vi "CSMLS - Continuous Loop in CSM Example.vi"() -> ()   [LabVIEW 2014]
uses:
  user.lib/_NEVSTOP/Communicable State Machine(CSM)/_Support/Priority Queue/Priority Queue.lvclass/Priority Queue.ctl
  user.lib/_NEVSTOP/Communicable State Machine(CSM)/_Support/Process/CSMP-Async Call.vi
  user.lib/_NEVSTOP/Communicable State Machine(CSM)/_Support/GlobalEvent/GEvt-Generate Status Log.vi
  user.lib/_NEVSTOP/Communicable State Machine(CSM)/_Support/Process/CSMP-Broadcast.vi
  user.lib/_NEVSTOP/Communicable State Machine(CSM)/_Support/GlobalEvent/GEvt-Generate Interrupt Log.vi
  user.lib/_NEVSTOP/Communicable State Machine(CSM)/_Support/GlobalEvent/GEvt-Generate Register Log.vi
  user.lib/_NEVSTOP/Communicable State Machine(CSM)/_Support/Process/CSMP-Register Status.vi
  user.lib/_NEVSTOP/Communicable State Machine(CSM)/_Support/GlobalEvent/GEvt-Generate Unregister Log.vi
  user.lib/_NEVSTOP/Communicable State Machine(CSM)/_Support/Process/CSMP-Unregister Status.vi
  user.lib/_NEVSTOP/Communicable State Machine(CSM)/_Support/Process/CSMP-Sync Call.vi
  user.lib/_NEVSTOP/Communicable State Machine(CSM)/_Support/CSMQ/_CSMObj-Unlock.vi
  user.lib/_NEVSTOP/Communicable State Machine(CSM)/_Support/Process/CSMP-PostPostMsg.vi
  user.lib/_NEVSTOP/Communicable State Machine(CSM)/_Support/Process/CSMP-PostSendMsg.vi
  user.lib/_NEVSTOP/Communicable State Machine(CSM)/_Support/CSMQ/_CSMObj-Lock State.vi
  user.lib/_NEVSTOP/Communicable State Machine(CSM)/_Support/Common/Splite Reason String Part.vi
  user.lib/_NEVSTOP/Communicable State Machine(CSM)/_Support/Common/Trim Single line Text.vi
  user.lib/_NEVSTOP/Communicable State Machine(CSM)/_Support/CSMQ/_CSMOFGV Release.vi
  user.lib/_NEVSTOP/Communicable State Machine(CSM)/_Support/Common/Remove Comments from Line.vi
  user.lib/_NEVSTOP/Communicable State Machine(CSM)/_Support/Common/Splite Single-line Message.vi
  user.lib/_NEVSTOP/Communicable State Machine(CSM)/_Support/Common/Parse Next Single-line State.vi
  user.lib/_NEVSTOP/Communicable State Machine(CSM)/_Support/CSMQ/_CSMOFGV Dequeue.vi
  user.lib/_NEVSTOP/Communicable State Machine(CSM)/_Support/CSMQ/_CSMObj-Log Error if in a Remote Session.vi
  user.lib/_NEVSTOP/Communicable State Machine(CSM)/_Support/GlobalEvent/GEvt-Generate State Change Log.vi
  user.lib/_NEVSTOP/Communicable State Machine(CSM)/_Support/GlobalEvent/GEvt-Generate Remaining States Log.vi
  user.lib/_NEVSTOP/Communicable State Machine(CSM)/_Support/GlobalEvent/GEvt-Generate Module Destroyed Log.vi
  user.lib/_NEVSTOP/Communicable State Machine(CSM)/_Support/GlobalEvent/GEvt-Generate Complete Log.vi
  user.lib/_NEVSTOP/Communicable State Machine(CSM)/_Support/GlobalEvent/GEvt-Generate Module Created Log.vi
  user.lib/_NEVSTOP/Communicable State Machine(CSM)/AdvanceAPI/CSM - Revert Arguments-Safe String.vi
  user.lib/_NEVSTOP/Communicable State Machine(CSM)/AdvanceAPI/CSM - Make String Arguments Safe.vi
  user.lib/_NEVSTOP/Communicable State Machine(CSM)/_Support/CSMQ/_CSMObj-Message Check.vi
  user.lib/_NEVSTOP/Communicable State Machine(CSM)/_Support/CSMQ/_CSMObj-Enqueue Cross-Module Message.vi
  user.lib/_NEVSTOP/Communicable State Machine(CSM)/_Support/CSMQ/_CSMOFGV Get.vi
  user.lib/_NEVSTOP/Communicable State Machine(CSM)/_Support/FGV-BroadcastRegistry/Cache-Broadcast Registry Search Result.vi
  user.lib/_NEVSTOP/Communicable State Machine(CSM)/AdvanceAPI/CSM - Register Status Change.vi
  user.lib/_NEVSTOP/Communicable State Machine(CSM)/AdvanceAPI/CSM - Unregister Status Change.vi
  user.lib/_NEVSTOP/Communicable State Machine(CSM)/_Support/Common/Hex Str to U8 Data.vi
  user.lib/_NEVSTOP/Communicable State Machine(CSM)/_Support/Common/Concatenate State with Arguments.vi
  user.lib/_NEVSTOP/Communicable State Machine(CSM)/_Support/Common/U8 Data to Hex Str.vi
  user.lib/_NEVSTOP/Communicable State Machine(CSM)/_Support/Priority Queue/Dequeue Element.vi
  user.lib/_NEVSTOP/Communicable State Machine(CSM)/AdvanceAPI/CSM - Keywords.vi
  user.lib/_NEVSTOP/Communicable State Machine(CSM)/_Support/Priority Queue/Enqueue Element.vi
  user.lib/_NEVSTOP/Communicable State Machine(CSM)/Utility/Trim Both Whitespace.vi
  user.lib/_NEVSTOP/Communicable State Machine(CSM)/_Support/GlobalEvent/FGV-GlobalEventRef.vi
  user.lib/_NEVSTOP/Communicable State Machine(CSM)/_Support/CSMQ/_CSMOFGV Obtain.vi
  user.lib/_NEVSTOP/Communicable State Machine(CSM)/_Support/CSMQ/_CSMOFGV.vi
  user.lib/_NEVSTOP/Communicable State Machine(CSM)/_Support/GlobalEvent/FGV-StatusChangeEventRef.vi
  user.lib/_NEVSTOP/Communicable State Machine(CSM)/_Support/FGV-BroadcastRegistry/global-Broadcast Cache Change Flag.vi
  user.lib/_NEVSTOP/Communicable State Machine(CSM)/_Support/FGV-BroadcastRegistry/FGV-BroadcastRegistry.vi
  user.lib/_NEVSTOP/Communicable State Machine(CSM)/Communicable State Machine.lvlib
  user.lib/_NEVSTOP/Communicable State Machine(CSM)/addons/Loop-Support/CSM Loop Support.lvlib
panel:
  in  "High-Priority Error":bool
  in  "Low-Priority Error":bool
  out "Filtered UI States":string
  out "UI States":string
  out ">> Source CSM >>":string
  out "Remaining States":string
  in  "DAQ: Once":bool
  out "Waveform Chart":dbl(graph)=7.7472539242125515
  in  "Center":dbl(slide) scale=0.0..10.0
  in  "Stop":bool
  in  "Start":bool
  out "State History":string
  in  "Name(\"\" to use uuid)":string="CSM Tiny"
  in  "Init State(\"Macro: Initialize\")":string="Macro: Initialize"
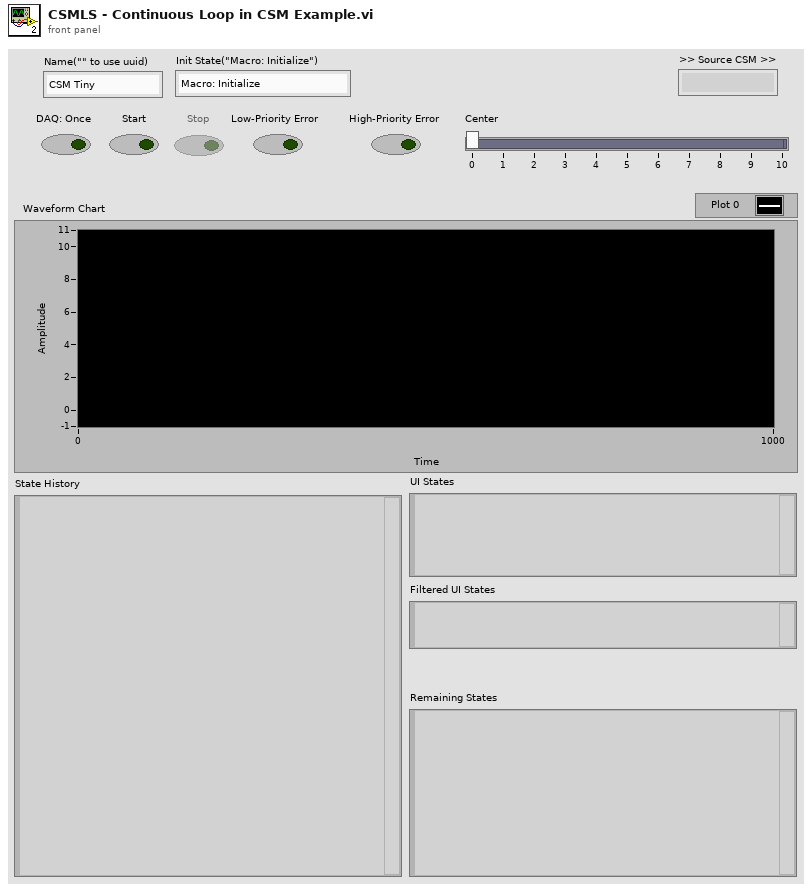
[diagram p1: front panel]
types:
  T1 = enum32{"Invalid", "Standard", "Closed", "Hidden", "Minimized", "Maximized"}
  T2 = enum32{"invalid app kind", "Development System", "Run Time System", "Student Edition", "Embedded LabVIEW", "Evaluation", "Custom"}
  T3 = typedef "Communicable State Machine.lvlib/_CSM_Response Source Message.ctl" = cluster{"‘State":string, "’Arguments":string, "’Error":errorcluster}
  T4 = cluster{"Core":cluster{"Current VI Reference":refnum<vi>, "Close Panel on Exit?":bool}, "IsRunning?":bool, "Center":dbl}
  T5 = cluster{"Current VI Reference":refnum<vi>, "Close Panel on Exit?":bool}
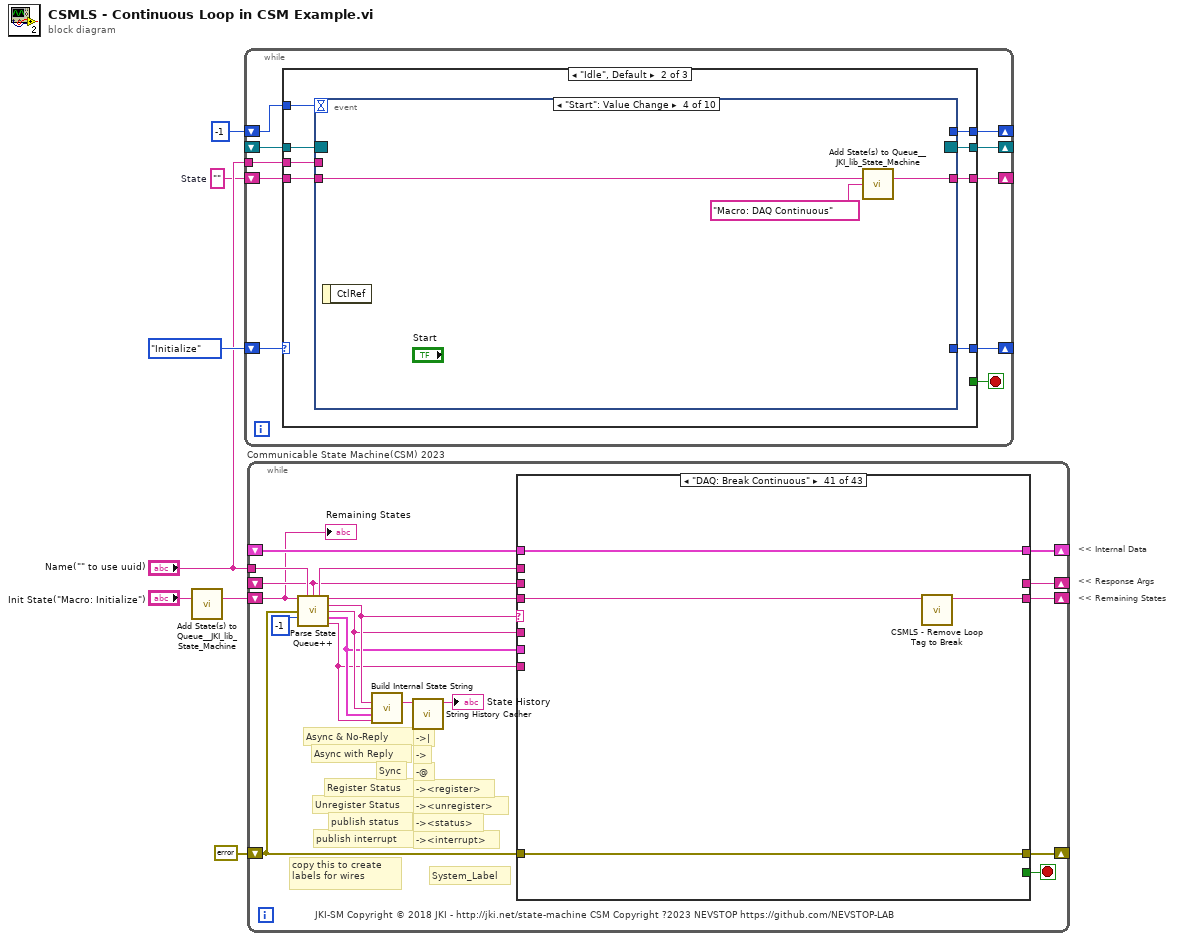
[diagram p0: block diagram]
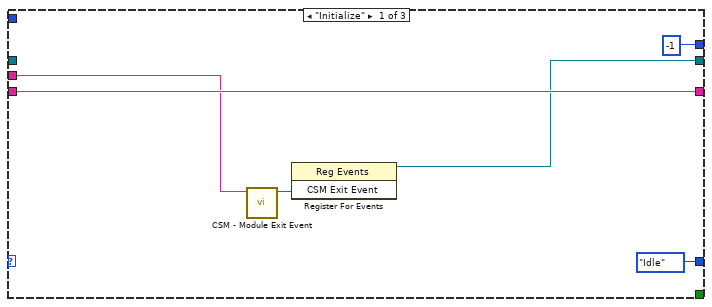
[diagram p2: hidden frame]
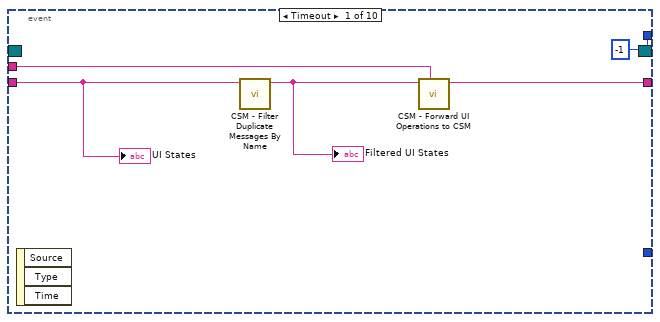
[diagram p3: hidden frame]
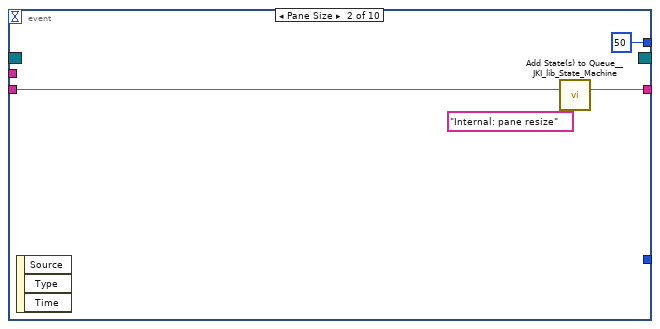
[diagram p4: hidden frame]
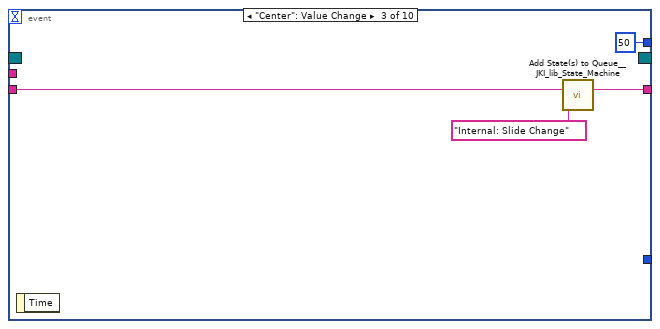
[diagram p5: hidden frame]
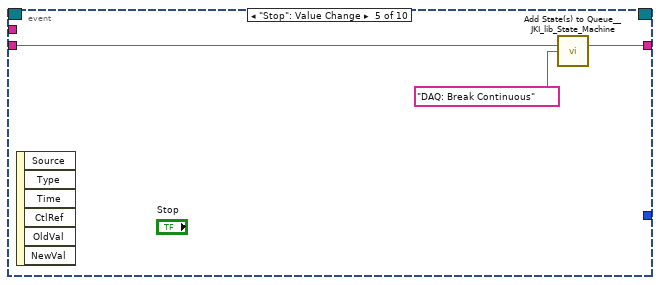
[diagram p6: hidden frame]
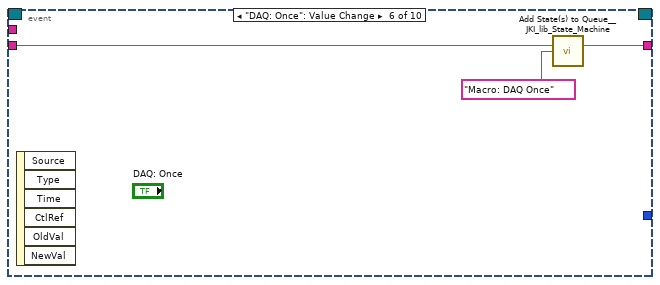
[diagram p7: hidden frame]
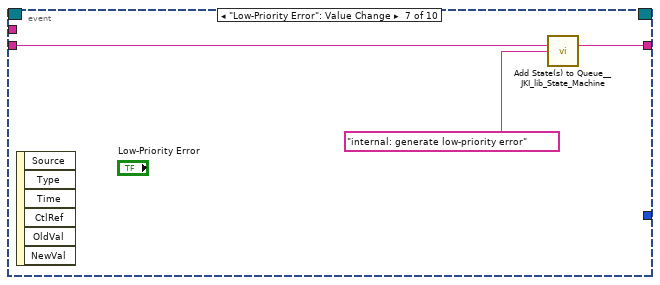
[diagram p8: hidden frame]
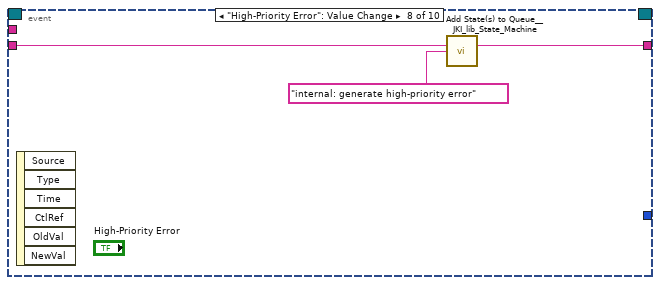
[diagram p9: hidden frame]
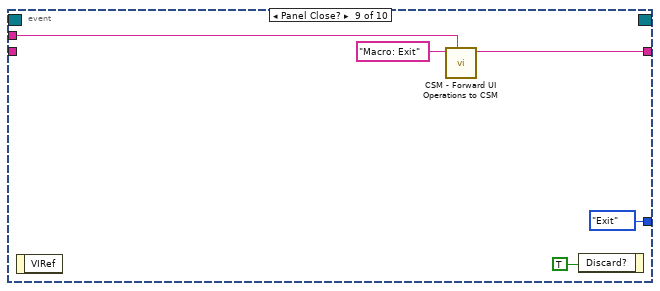
[diagram p10: hidden frame]
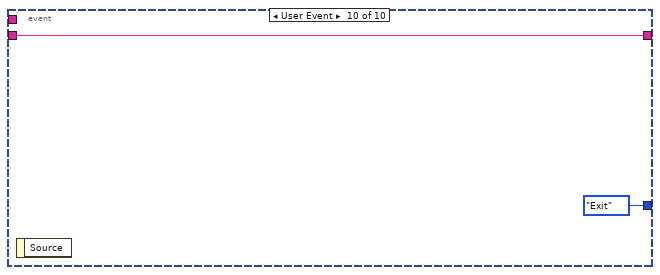
[diagram p11: hidden frame]
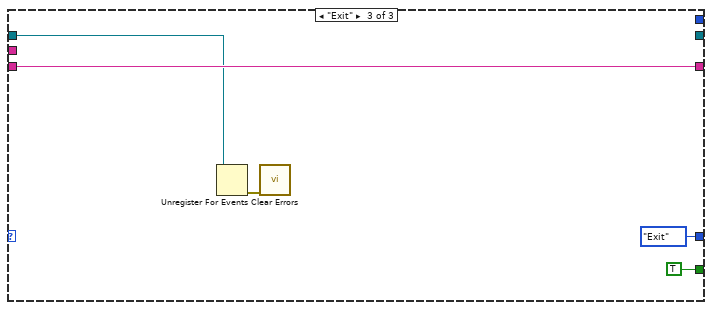
[diagram p12: hidden frame]
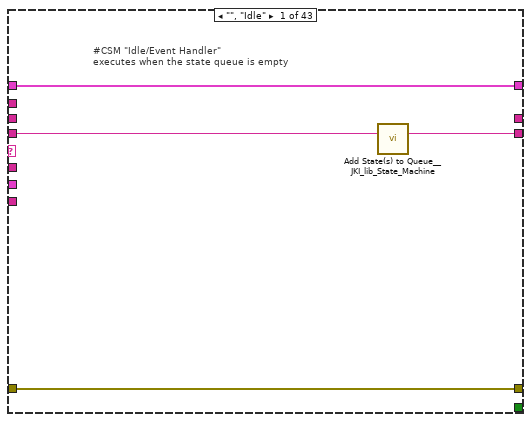
[diagram p13: hidden frame]
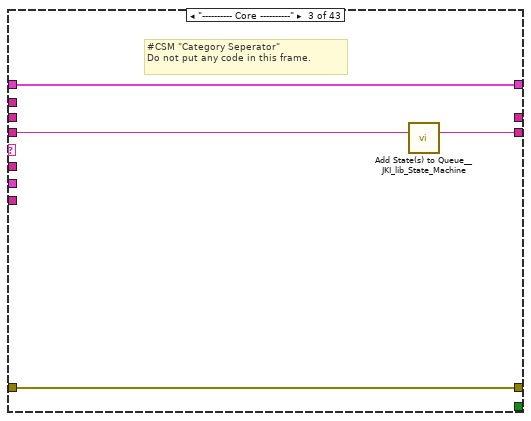
[diagram p15: hidden frame]
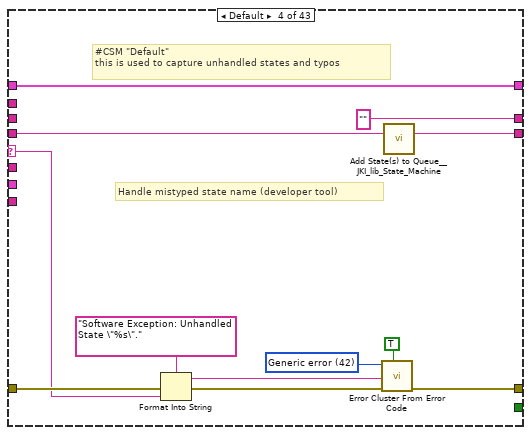
[diagram p16: hidden frame]
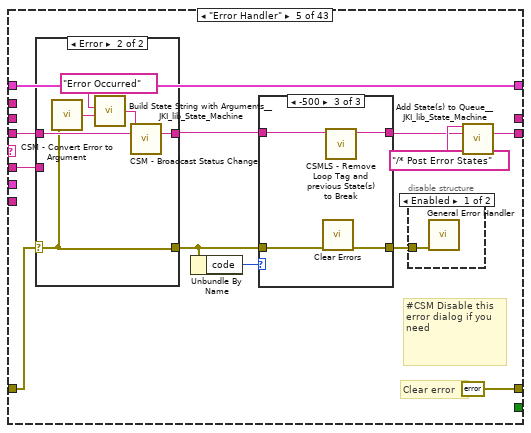
[diagram p17: hidden frame]
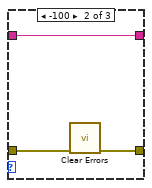
[diagram p19: hidden frame]
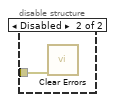
[diagram p20: hidden frame]
diagram:
  w2 = ""  # State
  # "<< Internal Data"
  # "<< Response Args"
  # "<< Remaining States"
  n1 = call <vilib>:"Add State(s) to Queue__JKI_lib_State_Machine.vi"("State(s) in (\"\")"="Init State(\"Macro: Initialize\")") -> ("States Out"=w5:string)  [unwired: 14 in]
  n2 = while {
    shift-right: [w16] -> _
    shift-left: enum16{"Idle", "Initialize", "Exit"}."Initialize" -> [w17]
    tunnel: "Name(\"\" to use uuid)" -> [w14]
    shift-right: [w12] -> _
    shift-left: w2 -> [w13]
    shift-right: [w10] -> _
    shift-left: -1 -> [w11]
    shift-right: [w9] -> _
    shift-left: _ -> [w8]
    stop <- w15 stop-if-true
    n3 = case shown="\"Idle\", Default" w17 {
      tunnel: [enum16{"Idle", "Initialize", "Exit"}."Idle" w31 enum16{"Idle", "Initialize", "Exit"}."Exit"] -> w16
      tunnel: [_ _ TRUE] -> w15
      tunnel: w14 -> [w19 w30 _]
      tunnel: w13 -> [w22 w28 w69]
      tunnel: [w22 w29 w69] -> w12
      tunnel: w11 -> [_ w26 _]
      tunnel: [-1 w27 _] -> w10
      tunnel: [w18 w24 _] -> w9
      tunnel: w8 -> [_ w25 w68]
      frame "Initialize" {
        n4 = call "CSM - Module Exit Event.vi"("Name(\"\" to use uuid) in"=w19) -> ("CSM Exit Event"=w20:refnum<user-event>)  [unwired: 9 in, 1 out]
        n5 = register-events(w20) -> (reference out=w18:refnum<event-registration>)  [unwired: 2 in, 1 out]
      }
      frame "Idle", Default {
        n6 = event shown="[3] \"Start\": Value Change" {
          selector: w25 -> [_ _ _ _ _ _ _ _ _ _]
          dyn-events: [_ _ _ _ _ _ _ _ _ _] -> w24
          timeout: w26 -> [_ _ _ _ _ _ _ _ _ _]
          tunnel: [_ _ _ _ _ _ _ _ enum16{"Idle", "Initialize", "Exit"}."Exit" enum16{"Idle", "Initialize", "Exit"}."Exit"] -> w31
          tunnel: w30 -> [w32 _ _ _ _ _ _ _ w61 _]
          tunnel: w28 -> [w35 w40 w44 w47 w49 w52 w56 w58 _ w66]
          tunnel: [w33 w39 w43 w46 w50 w53 w55 w57 w60 w66] -> w29
          tunnel: [-1 50 50 _ _ _ _ _ _ _] -> w27
          event Timeout {
            n7 = event-data() -> ()  [unwired: 1 in, 3 out]
            n8 = call "CSM - Filter Duplicate Messages By Name.vi"("States"=w35) -> ("States out"=w34:string)  [unwired: 10 in]
            "Filtered UI States" <- w34
            n9 = call "CSM - Forward UI Operations to CSM.vi"("Name(\"\" to use uuid)"=w32, "State(s) in (\"\")"=w34) -> ("States Out"=w33:string)  [unwired: 9 in]
            "UI States" <- w35
          }
          event Pane Size {
            n10 = event-data() -> ()  [unwired: 1 in, 3 out]
            n11 = call <vilib>:"Add State(s) to Queue__JKI_lib_State_Machine.vi"("State(s) in (\"\")"=w40, "State(s) at Back (\"\")"="Internal: pane resize" ("State(s) at Back (\"\")")) -> ("States Out"=w39:string)  [unwired: 13 in]
          }
          event "Center": Value Change {
            n12 = event-data() -> ()  [unwired: 1 in, 1 out]
            n13 = call <vilib>:"Add State(s) to Queue__JKI_lib_State_Machine.vi"("State(s) in (\"\")"=w44, "State(s) at Back (\"\")"="Internal: Slide Change" ("State(s) at Back (\"\")")) -> ("States Out"=w43:string)  [unwired: 13 in]
          }
          event "Start": Value Change {
            n14 = event-data() -> ()  [unwired: 1 in, 1 out]
            n15 = call <vilib>:"Add State(s) to Queue__JKI_lib_State_Machine.vi"("State(s) in (\"\")"=w47, "State(s) at Back (\"\")"="Macro: DAQ Continuous" ("State(s) at Back (\"\")")) -> ("States Out"=w46:string)  [unwired: 13 in]
          }
          event "Stop": Value Change {
            n16 = event-data() -> ()  [unwired: 1 in, 6 out]
            n17 = call <vilib>:"Add State(s) to Queue__JKI_lib_State_Machine.vi"("State(s) in (\"\")"=w49, "State(s) at Back (\"\")"="DAQ: Break Continuous" ("State(s) at Back (\"\")")) -> ("States Out"=w50:string)  [unwired: 13 in]
          }
          event "DAQ: Once": Value Change {
            n18 = event-data() -> ()  [unwired: 1 in, 6 out]
            n19 = call <vilib>:"Add State(s) to Queue__JKI_lib_State_Machine.vi"("State(s) in (\"\")"=w52, "State(s) at Back (\"\")"="Macro: DAQ Once" ("State(s) at Back (\"\")")) -> ("States Out"=w53:string)  [unwired: 13 in]
          }
          event "Low-Priority Error": Value Change {
            n20 = event-data() -> ()  [unwired: 1 in, 6 out]
            n21 = call <vilib>:"Add State(s) to Queue__JKI_lib_State_Machine.vi"("State(s) in (\"\")"=w56, "State(s) at Back (\"\")"="internal: generate low-priority error" ("State(s) at Back (\"\")")) -> ("States Out"=w55:string)  [unwired: 13 in]
          }
          event "High-Priority Error": Value Change {
            n22 = event-data() -> ()  [unwired: 1 in, 6 out]
            n23 = call <vilib>:"Add State(s) to Queue__JKI_lib_State_Machine.vi"("State(s) in (\"\")"=w58, "State(s) at Back (\"\")"="internal: generate high-priority error" ("State(s) at Back (\"\")")) -> ("States Out"=w57:string)  [unwired: 13 in]
          }
          event Panel Close? {
            n24 = event-data() -> ()  [unwired: 1 in, 1 out]
            n25 = call "CSM - Forward UI Operations to CSM.vi"("Name(\"\" to use uuid)"=w61, "State(s) in (\"\")"="Macro: Exit" ("State")) -> ("States Out"=w60:string)  [unwired: 9 in]
            n26 = event-data("Discard?"=TRUE) -> ()  [unwired: 1 in, 1 out]
          }
          event User Event {
            n27 = event-data() -> ()  [unwired: 1 in, 1 out]
          }
        }
      }
      frame "Exit" {
        n28 = Unregister For Events(event registration refnum=w68) -> (error out=w67:errorcluster)  [unwired: 1 in]
        n29 = call <vilib>:"Clear Errors.vi"("error in (no error)"=w67) -> ()  [unwired: 5 in, 2 out]
      }
    }
  }
  n30 = while "Communicable State Machine(CSM) 2023" {
    shift-right: [w86] -> _
    shift-left: _ -> [w85]
    shift-right: [w89] -> _
    shift-left: errorcluster {"status"=FALSE, "code"=0, "source"=""} ("error out") -> [w84]
    shift-right: [w88] -> _
    shift-left: w5 -> [w72]
    tunnel: "Name(\"\" to use uuid)" -> [w82]
    shift-right: [w83] -> _
    shift-left: _ -> [w74]
    stop <- w87 stop-if-true
    # "-><interrupt>"
    # "-><status>"
    # "-><unregister>"
    # "-><register>"
    # "-@"
    # "->"
    # "->|"
    # "publish interrupt"
    # "publish status"
    # "Unregister Status"
    # "Register Status"
    # "Sync"
    # "Async with Reply"
    # "Async & No-Reply"
    # "copy this to create labels for wires"
    # "System_Label"
    # "JKI-SM Copyright © 2018 JKI - http://jki.net/state-machine CSM Copyright ?2023 NEVSTOP https://github.com/NEVSTOP-LAB"
    n31 = call "Parse State Queue++.vi"("State Queue"=w72, "Name(\"\" to use uuid)"=w82, "Response Arguments"=w74, "Error In (no error)"=w84, "Dequeue Timeout(0ms)"=-1 ("Timeout")) -> ("Name Used"=w75:string, "Remaining States"=w90:string, "Current State"=w79:string, "Arguments"=w78:string, ">> Response Source Message >>"=w77:T3, ">> Source CSM >>"=w76:string)  [unwired: 5 in]
    n32 = call "Build Internal State String.vi"("State"=w79, "Arguments (\"\")"=w78, ">> Response Source Message >>"=w77, "Source (\"\")"=w76) -> ("State with Arguments"=w80:string)  [unwired: 11 in]
    n33 = call "String History Cacher.vi"("String"=w80) -> ("String Cache"=→"State History":string)  [unwired: 10 in]
    n34 = case shown="\"DAQ: Break Continuous\"" w79 {
      selector: w79 -> [_ _ _ w103 _ _ w160 _ _ _ _ _ _ _ _ _ _ _ _ _ _ _ _ _ _ _ _ _ _ _ _ _ _ _ _ _ _ _ _ w417 _ _ _]
      tunnel: w90 -> [w91 w96 w101 w107 w122 w154 w162 w172 w183 w197 w202 w206 w213 w215 w222 w226 w232 w238 w253 w331 w336 w341 w343 w348 w352 w360 w364 w369 w376 w380 w384 w388 w392 w395 w397 w400 w403 w408 w414 w419 w425 w431 w434]
      tunnel: w78 -> [_ _ _ _ w121 w147 w161 w171 _ _ _ _ _ _ _ _ _ w233 w247 _ _ _ _ _ _ _ _ w367 _ _ _ _ _ _ _ _ _ _ _ _ _ _ _]
      tunnel: w85 -> [w92 w95 w98 w105 w124 w155 w163 w174 w182 w190 w200 w203 _ w214 w217 w223 w230 w236 w249 w330 w333 w338 w345 w350 w354 w359 w363 w368 w373 w377 w381 w387 w391 w394 w396 w399 w402 w407 w411 w422 w426 w430 w433]
      tunnel: [w93 w97 w99 w109 errorcluster {"status"=FALSE, "code"=0, "source"=""} ("error out") w156 w158 w177 w184 w194 w199 w204 w210 w216 w218 w224 w229 w234 w250 w332 w334 w339 w346 w351 w357 w361 w365 w370 w374 w378 w382 w389 errorcluster {"status"=TRUE, "code"=-100, "source"="Low priority error. Daq could continue."} ("error out") errorcluster {"status"=TRUE, "code"=-500, "source"="High priority error. Daq need stop!"} ("error out") w398 w401 w404 w409 w415 w423 w427 w432 w435] -> w89
      tunnel: w84 -> [w93 w97 w99 w108 w123 w156 w165 _ w184 w194 w199 w204 w210 w216 w219 w224 w229 w235 w251 w332 w334 w339 w346 w351 w357 w361 w365 w370 w374 w378 w382 w389 _ _ w398 w401 w404 w409 w415 w423 w427 w432 w435]
      tunnel: [w94 w96 w100 w106 w119 w153 w164 w173 w183 w196 w201 w205 w212 w215 w221 w225 w231 w237 w252 w331 w335 w340 w344 w349 w358 w360 w364 w369 w375 w379 w383 w388 w392 w395 w397 w400 w403 w408 w414 w420 w424 w431 w434] -> w88
      tunnel: [_ _ _ _ _ TRUE _ _ _ _ TRUE _ _ _ _ _ _ _ _ _ _ _ _ _ _ _ _ _ _ _ _ _ _ _ _ _ _ _ _ _ _ _ _] -> w87
      tunnel: [w92 w95 w98 w105 w124 w155 w163 w175 w182 w195 w200 w203 w211 w214 w217 w223 w230 w236 w249 w330 w333 w338 w345 w350 w354 w359 w363 w368 w373 w377 w381 w386 w391 w394 w396 w399 w402 w406 w411 w422 w426 w429 w433] -> w86
      tunnel: w76 -> [_ _ _ _ _ _ _ w169 _ _ _ _ _ _ _ _ _ _ _ _ _ _ _ _ _ _ _ _ _ _ _ _ _ _ _ _ _ _ _ w418 _ _ _]
      tunnel: w77 -> [_ _ _ _ _ _ _ w176 _ _ _ _ _ _ _ _ _ _ _ _ _ _ _ _ _ _ _ _ _ _ _ _ _ _ _ _ _ _ _ _ _ _ _]
      tunnel: [_ _ _ "" _ _ _ _ _ _ _ _ _ _ _ _ _ _ _ _ _ _ _ _ _ _ "API1 Response" w366 _ _ _ _ _ _ _ _ _ _ _ _ _ _ _] -> w83
      tunnel: w75 -> [_ _ _ _ _ _ _ _ _ _ _ _ _ _ _ _ _ _ _ _ _ _ _ _ _ _ _ _ _ _ _ _ _ _ _ _ _ _ _ _ _ _ _]
      tunnel: w74 -> [_ _ _ _ _ _ _ _ _ _ _ _ _ _ _ _ _ _ _ _ _ _ _ _ _ _ _ _ _ _ _ _ _ _ _ _ _ _ _ _ _ _ _]
      frame "", "Idle" {
        # "#CSM \"Idle/Event Handler\"\nexecutes when the state queue is empty"
        n35 = call <vilib>:"Add State(s) to Queue__JKI_lib_State_Machine.vi"("State(s) in (\"\")"=w91) -> ("States Out"=w94:string)  [unwired: 14 in]
      }
      frame "CSM Documentation" {
        # "#CSM README FIRST\n\nCSM is a LabVIEW application framework that builds upon JKI State Machine (JKISM). It follows the pattern of JKISM and extends the keywords to describe message communication between CSM modules, including concepts such as Sync-Message, Async-Message, Subscription/Unsubscription of status - essential elements for creating reusable code modules. For more information, please visit the CSM wiki: https://github.com/NEVSTOP-LAB/JKI-State-Machine-Plus-Plus/wiki\n\nFor instructions on JKI State Machine, visit: http://jki.net/state-machine/\nFor information about CSM, visit: https://github.com/NEVSTOP-LAB"
        # "#CSM \"Documentation\"\nCase for holding CSM Documenation"
      }
      frame "---------- Core ----------" {
        # "#CSM \"Category Seperator\"\nDo not put any code in this frame."
        n36 = call <vilib>:"Add State(s) to Queue__JKI_lib_State_Machine.vi"("State(s) in (\"\")"=w101) -> ("States Out"=w100:string)  [unwired: 14 in]
      }
      frame Default {
        w112 = 42 items=["No error", "Argument error", "Memory is full", "Out of zone", "End of file", "File already open", "Generic file I/O error", "File not found", "File permission error", "Disk is full", "Duplicate path", "Too many files open", "System feature not enabled", "Resource file not found", "Cannot add resource", "Resource not found", "Image not found", "Image memory error", "Pen does not exist", "Config type invalid", "Config token not found", "Config parse error", "Config memory error", "Bad external code format", "Bad external code offset", "External code not present", "Null window", "Destroy window error", "Null menu", "Print aborted", "Bad print record", "Print driver error", "Windows error during printing", "Memory error during printing", "Print dialog error", "Generic print error", "Invalid device refnum", "Device not found", "Device parameter error", "Device unit error", "Cannot open device", "Device call aborted", "Generic error", "Cancelled by user", "Object ID too low", "Object ID too high", "Object not in heap", "Unknown heap", "Unknown object (invalid DefProc)", "Unknown object (DefProc not in table)", "Message out of range", "Invalid (null) method", "Unknown message", "Manager call not supported", "Bad address", "Network operation in progress", "Network operation timed out", "Connection is busy", "Network attribute not supported", "Network error", "Address in use", "System out of memory", "Connection aborted", "Connection refused", "Not connected", "Already connected", "Connection closed", "Initialization error (interapplication manager)", "Bad occurrence", "Wait on unbound occurrence handler", "Occurrence queue overflow", "Datalog type conflict", "Unused", "Unrecognized type (interapplication manager)", "Memory corrupt", "Failed to make temporary DLL", "Old CIN version", "Drag socket not found", "Failed to load drop-object", "Failed to register OLE object", "Failed to release OLE object", "Format specifier type mismatch", "Unknown format specifier", "Too few format specifiers", "Too many format specifiers", "Scan failed", "Newer CIN version", "Error converting to variant", "Runtime menu error", "Password tampered", "Variant attribute not found", "Incompatible variant data type", "Event data is not available", "Event Store is not present", "Occurrence is not found", "Event Queue is not created", "Event info is not available", "Refnum passed is NULL", "Error retrieving Class GUID", "Error retrieving CoClass GUID", "Error retrieving TypeLib GUID.", "Bad built application magic bytes.", "Specific driver is different from the specific driver associated with the Logical Name.", "There is no session opened to the class driver.", "Max Error", "MAX - Error with config objects", "MAX - Error loading configuration", "MAX - Group not supported"]
        # "#CSM \"Default\"\nthis is used to capture unhandled states and typos"
        # "Handle mistyped state name (developer tool)"
        n37 = Format Into String(format string="Software Exception: Unhandled State \"%s\"." ("message"), error in=w108, w103) -> (resulting string=w111:string, error out=w110:errorcluster)  [unwired: 1 in]
        n38 = call <vilib>:"Error Cluster From Error Code.vi"("show call chain? (False)"=TRUE, "error in (no error)"=w110, "error message (\"\")"=w111, "error code (0)"=w112) -> ("error out"=w109:errorcluster)  [unwired: 5 in]
        n39 = call <vilib>:"Add State(s) to Queue__JKI_lib_State_Machine.vi"("State(s) in (\"\")"=w107) -> ("States Out"=w106:string)  [unwired: 14 in]
      }
      frame "Error Handler" {
        # "#CSM Disable this error dialog if you need"
        # "Clear error"
        n40 = case shown="Error" w123 {
          selector: w123 -> [_ w140]
          tunnel: [w139 w141] -> w114
          tunnel: w122 -> [w139 w142]
          tunnel: w121 -> [w138 _]
          tunnel: [w137 w140] -> w117
          frame No Error {
            n41 = call "CSM - Convert Argument to Error.vi"("Argument"=w138) -> ("error"=w137:errorcluster)  [unwired: 4 in]
          }
          frame Error {
            n42 = call "CSM - Convert Error to Argument.vi"("error in (no error)"=w140) -> ("Arguments"=w144:string)  [unwired: 4 in]
            n43 = call <vilib>:"Build State String with Arguments__JKI_lib_State_Machine.vi"("Arguments (\"\")"=w144, "State"="Error Occurred" ("Status with Arguments")) -> ("State with Arguments"=w143:string)  [unwired: 4 in]
            n44 = call "CSM - Broadcast Status Change.vi"("Status with Arguments"=w143, "State Queue"=w142) -> ("Remaining States"=w141:string)  [unwired: 13 in]
          }
        }
        n45 = Unbundle By Name(w117) -> ("code"=w118:i32)
        n46 = case shown="-500" w118 {
          tunnel: w117 -> [w127 w130 w134]
          tunnel: [w127 w129 w131] -> w116
          tunnel: [w126 w128 w132] -> w115
          tunnel: w114 -> [w126 w128 w133]
          frame 0, Default {
          }
          frame -100 {
            n47 = call <vilib>:"Clear Errors.vi"("error in (no error)"=w130) -> ("error out"=w129:errorcluster)  [unwired: 5 in, 1 out]
          }
          frame -500 {
            n48 = call <vilib>:"Clear Errors.vi"("error in (no error)"=w134) -> ("error out"=w131:errorcluster)  [unwired: 5 in, 1 out]
            n49 = call "CSMLS - Remove Loop Tag and previous State(s) to Break.vi"("Remaining States"=w133) -> ("States"=w132:string)  [unwired: 10 in]
          }
        }
        n50 = disable-structure shown="Enabled" {
          disable-tunnel: w116 -> [w135 w136]
          frame Enabled {
            n51 = call <vilib>:"General Error Handler.vi"("error in (no error)"=w135) -> ()  [unwired: 10 in, 5 out]
          }
          frame Disabled {
            n52 = call <vilib>:"Clear Errors.vi"("error in (no error)"=w136) -> ()  [unwired: 5 in, 2 out]
          }
        }
        n53 = call <vilib>:"Add State(s) to Queue__JKI_lib_State_Machine.vi"("State(s) in Front (\"\")"="/* Post Error States", "State(s) in (\"\")"=w115) -> ("States Out"=w119:string)  [unwired: 13 in]
      }
      frame "Critical Error" {
        w151 = 42 items=["No error", "Argument error", "Memory is full", "Out of zone", "End of file", "File already open", "Generic file I/O error", "File not found", "File permission error", "Disk is full", "Duplicate path", "Too many files open", "System feature not enabled", "Resource file not found", "Cannot add resource", "Resource not found", "Image not found", "Image memory error", "Pen does not exist", "Config type invalid", "Config token not found", "Config parse error", "Config memory error", "Bad external code format", "Bad external code offset", "External code not present", "Null window", "Destroy window error", "Null menu", "Print aborted", "Bad print record", "Print driver error", "Windows error during printing", "Memory error during printing", "Print dialog error", "Generic print error", "Invalid device refnum", "Device not found", "Device parameter error", "Device unit error", "Cannot open device", "Device call aborted", "Generic error", "Cancelled by user", "Object ID too low", "Object ID too high", "Object not in heap", "Unknown heap", "Unknown object (invalid DefProc)", "Unknown object (DefProc not in table)", "Message out of range", "Invalid (null) method", "Unknown message", "Manager call not supported", "Bad address", "Network operation in progress", "Network operation timed out", "Connection is busy", "Network attribute not supported", "Network error", "Address in use", "System out of memory", "Connection aborted", "Connection refused", "Not connected", "Already connected", "Connection closed", "Initialization error (interapplication manager)", "Bad occurrence", "Wait on unbound occurrence handler", "Occurrence queue overflow", "Datalog type conflict", "Unused", "Unrecognized type (interapplication manager)", "Memory corrupt", "Failed to make temporary DLL", "Old CIN version", "Drag socket not found", "Failed to load drop-object", "Failed to register OLE object", "Failed to release OLE object", "Format specifier type mismatch", "Unknown format specifier", "Too few format specifiers", "Too many format specifiers", "Scan failed", "Newer CIN version", "Error converting to variant", "Runtime menu error", "Password tampered", "Variant attribute not found", "Incompatible variant data type", "Event data is not available", "Event Store is not present", "Occurrence is not found", "Event Queue is not created", "Event info is not available", "Refnum passed is NULL", "Error retrieving Class GUID", "Error retrieving CoClass GUID", "Error retrieving TypeLib GUID.", "Bad built application magic bytes.", "Specific driver is different from the specific driver associated with the Logical Name.", "There is no session opened to the class driver.", "Max Error", "MAX - Error with config objects", "MAX - Error loading configuration", "MAX - Group not supported"]
        # "#CSM Stop in Critical Error\nWhen Critical Error occurs, Stop the loop immediately. Do NOT change this unless you fully understand the impact."
        # "#CSM \"Critical Error\"\nWhen any un-recoverable error occurs, CSM goes into this case."
        # "Handle mistyped state name (developer tool)"
        n54 = Format Into String(format string="Software Exception: Critical Error\"%s\"." ("message"), w147) -> (resulting string=w150:string, error out=w149:errorcluster)  [unwired: 2 in]
        n55 = call <vilib>:"Error Cluster From Error Code.vi"("show call chain? (False)"=TRUE, "error in (no error)"=w149, "error message (\"\")"=w150, "error code (0)"=w151) -> ()  [unwired: 5 in, 1 out]
        n56 = call <vilib>:"Add State(s) to Queue__JKI_lib_State_Machine.vi"("State(s) in (\"\")"=w154) -> ("States Out"=w153:string)  [unwired: 14 in]
      }
      frame "Target Error", "Target Timeout Error" {
        # "#CSM \"Target Error\"\nWhen This CSM try to communicate with an un-existed CSM, This CSM goes into this case."
        # "#CSM \"Target Timeout Error\"\nWhen This CSM could not get the sync-call response in time, This CSM goes into this case."
        n57 = Format Into String(format string="Software Exception: %s now \"%s\"." ("message"), error in=w165, w160, w161) -> (resulting string=w159:string)  [unwired: 1 in, 1 out]
        n58 = call "Build Error Cluster.vi"("String to Prepend to source (\"\")"=w159, "code"=-1) -> ("error out"=w158:errorcluster)
        n59 = call <vilib>:"Add State(s) to Queue__JKI_lib_State_Machine.vi"("State(s) in (\"\")"=w162) -> ("States Out"=w164:string)  [unwired: 14 in]
      }
      frame "Async Response", "Response" {
        n60 = Unbundle(w176) -> ("‘State"=w170:string, "’Arguments"=w168:string, "’Error"=w167:errorcluster)
        n61 = case shown="Default" w170 {
          tunnel: [w181] -> w177
          tunnel: w167 -> [w181]
          tunnel: [w180] -> w175
          tunnel: w174 -> [w180]
          tunnel: [w178] -> w173
          tunnel: w172 -> [w179]
          tunnel: w171 -> [_]
          tunnel: w169 -> [_]
          tunnel: w168 -> [_]
          frame Default {
            # "#CSM Response Comments\nAfter Message is executed, CSM goes to this state for receive the response.\n    For Async Message(->), \"Async Response\" is used. This CSM will goes to \"Async Message Posted\" immediately and receive the \"Async Response\" after the callee finishes the message.\n    For Sync Message(@),  This CSM will wait until the message is done and immediately goes to \"Response\""
            # "#CSM \"Async Response\"\nHandle Async-call Response (\"Async Response\" for ->)"
            # "#CSM \"Response\"\nHandle Sync-call Response (\"Response\" for -@)"
            n62 = call <vilib>:"Add State(s) to Queue__JKI_lib_State_Machine.vi"("State(s) in (\"\")"=w179) -> ("States Out"=w178:string)  [unwired: 14 in]
          }
        }
      }
      frame "Async Message Posted" {
        # "#CSM \"Async Message Posted\"\nAfter Async Message is posted (-> or ->| ), CSM goes to this state for post-action.\nYou can use Argument - State to tell which Async Message is called."
      }
      frame "Initialize Core Data" {
        # "#CSM \"Initialize Core Data\"\nThis is used to determine panel behavior on exit"
        # "originally closed?"
        # "exe?"
        # "If panel starts closed or is an EXE, then close it when we exit"
        n63 = property class="VI"() -> ("FP.State"=w187:T1)  [unwired: 2 in, 2 out]
        n64 = property class="App"() -> ("App.Kind"=w193:T2)  [unwired: 2 in, 2 out]
        n65 = control-ref of="Current VI Reference"() -> (w188:refnum<vi>)
        n66 = Equal?(x=w187, y=T1."Closed" ("Front Panel Window:State")) -> (x = y?=w185:bool)
        n67 = Equal?(x=w193, y=T2."Run Time System" ("Application:Kind")) -> (x = y?=w191:bool)
        n68 = Or(x=w185, y=w191) -> (x .or. y?=w189:bool)
        n69 = Bundle By Name(cluster=w190, "Core.Current VI Reference"=w188, "Core.Close Panel on Exit?"=w189) -> (w195:T4)
        n70 = call <vilib>:"Add State(s) to Queue__JKI_lib_State_Machine.vi"("State(s) in (\"\")"=w197) -> ("States Out"=w196:string)  [unwired: 14 in]
      }
      frame "Exit" {
        # "#CSM \"Exit\"\nCase for exiting the loop. No errors that occur here will be handled."
        n71 = call <vilib>:"Add State(s) to Queue__JKI_lib_State_Machine.vi"("State(s) in (\"\")"=w202) -> ("States Out"=w201:string)  [unwired: 14 in]
      }
      frame "---------- Data ----------" {
        # "#CSM \"Category Seperator\"\nDo not put any code in this frame."
        n72 = call <vilib>:"Add State(s) to Queue__JKI_lib_State_Machine.vi"("State(s) in (\"\")"=w206) -> ("States Out"=w205:string)  [unwired: 14 in]
      }
      frame "Data: Initialize" {
        w208 = T5 {"Current VI Reference"=refnum, "Close Panel on Exit?"=FALSE}  # Core
        w209 = FALSE  # IsRunning?
        # "do not delete - used by framework"
        # "Expand Bundle to add new data elements to shift register data."
        # "Initialize the shift-register data, here.\n(data names are defined by what you wire into the bundle function)"
        n73 = local read "Center"() -> (w207:dbl)
        n74 = Bundle("Core"=w208, "IsRunning?"=w209, "Center"=w207) -> (w211:T4)  [unwired: 1 in]
        n75 = call <vilib>:"Add State(s) to Queue__JKI_lib_State_Machine.vi"("State(s) in (\"\")"=w213) -> ("States Out"=w212:string)  [unwired: 14 in]
      }
      frame "Data: Update Indicators" {
      }
      frame "Data: Cleanup" {
        # "Cleanup any data and references, here.\n(this is called automatically, by the Macro: Exit)"
        n76 = Unbundle By Name(w217) -> ("Core.Current VI Reference"=w220:refnum<vi>)
        n77 = Close Reference(reference=w220, error in (no error)=w219) -> (error out=w218:errorcluster)
        n78 = call <vilib>:"Add State(s) to Queue__JKI_lib_State_Machine.vi"("State(s) in (\"\")"=w222) -> ("States Out"=w221:string)  [unwired: 14 in]
      }
      frame "---------- UI ----------" {
        # "#CSM \"Category Seperator\"\nDo not put any code in this frame."
        n79 = call <vilib>:"Add State(s) to Queue__JKI_lib_State_Machine.vi"("State(s) in (\"\")"=w226) -> ("States Out"=w225:string)  [unwired: 14 in]
      }
      frame "UI: Initialize" {
        # "#CSM \"UI: Initialize\"\nInitialize the User Interface, here.\n(this is called automatically, by the Macro: Init)"
        n80 = property on="Waveform Chart" class="WFChart (strict)"("History Data"=dbl[] []) -> ()  [unwired: 2 in, 2 out]
        n81 = call <vilib>:"Add State(s) to Queue__JKI_lib_State_Machine.vi"("State(s) in Front (\"\")"="UI: Refresh Buttons" ("State(s) in Front (\"\")"), "State(s) in (\"\")"=w232) -> ("States Out"=w231:string)  [unwired: 13 in]
      }
      frame "UI: Cursor Set" {
        # "#CSM \"UI: Cursor Set\"\nSet and Unset Cursor Busy.\n(Usage: \"UI: Cursor Set >> Busy|Idle\")"
        # "Argument"
        n82 = disable-structure shown="TARGET_TYPE!=Windows" {
          disable-tunnel: w235 -> [w241 w246]
          disable-tunnel: [w240 w246] -> w234
          disable-tunnel: w233 -> [w239 _]
          frame condition #0 (active) {
            n83 = case shown="\"Idle\", Default" w239 {
              tunnel: w241 -> [w243 w245]
              tunnel: [w242 w244] -> w240
              frame "Idle", Default {
                n84 = call <vilib>:"Unset Busy.vi"("error in (no error)"=w243) -> ("error out"=w242:errorcluster)  [unwired: 10 in]
              }
              frame "Busy" {
                n85 = call <vilib>:"Set Busy.vi"("error in (no error)"=w245) -> ("error out"=w244:errorcluster)  [unwired: 9 in, 1 out]
              }
            }
          }
          frame condition #1 {
          }
        }
        n86 = call <vilib>:"Add State(s) to Queue__JKI_lib_State_Machine.vi"("State(s) in (\"\")"=w238) -> ("States Out"=w237:string)  [unwired: 14 in]
      }
      frame "UI: Front Panel State" {
        # "#CSM \"UI: Front Panel State\"\nSet Front Panel Open or Closed\n(Usage: \"UI: Front Panel State >> Open|Close\")"
        # "Argument"
        n87 = Unbundle By Name(w249) -> ("Core.Current VI Reference"=w248:refnum<vi>)
        n88 = call <vilib>:"Add State(s) to Queue__JKI_lib_State_Machine.vi"("State(s) in (\"\")"=w253) -> ("States Out"=w252:string)  [unwired: 14 in]
        n89 = case shown="\"Close\", \"Closed\"" w247 {
          tunnel: w251 -> [w259 w274 w285 w298 w311]
          tunnel: [w261 w275 w287 w300 w313] -> w250
          tunnel: w248 -> [w260 w272 w286 w299 w312]
          frame "Open", "Standard", Default {
            w254 = T1."Standard" ("State")
            n90 = property class="VI"(reference=w260, error in=w259) -> (reference out=w257:refnum<vi>, error out=w258:errorcluster, "FP.State"=w256:T1)
            n91 = Not Equal?(x=w256, y=w254) -> (x != y?=w255:bool)
            n92 = case shown="True" w255 {
              tunnel: [w265 w267] -> w261
              tunnel: w258 -> [w264 w267]
              tunnel: w257 -> [w263 _]
              tunnel: w254 -> [w262 _]
              frame True {
                n93 = invoke class="VI" method="FP.Open"(reference=w263, error in=w264, "Activate"=TRUE, "State"=w262) -> (error out=w265:errorcluster)  [unwired: 1 in, 4 out]
              }
              frame False {
              }
            }
          }
          frame "Close", "Closed" {
            n94 = property class="VI"(reference=w272, error in=w274) -> (reference out=w271:refnum<vi>, error out=w273:errorcluster, "FP.State"=w269:T1)
            n95 = Not Equal?(x=w269, y=T1."Closed" ("Front Panel Window:State")) -> (x != y?=w268:bool)
            n96 = case shown="False" w268 {
              tunnel: [w276 w279] -> w275
              tunnel: w273 -> [w276 w278]
              tunnel: w271 -> [_ w277]
              frame False {
              }
              frame True {
                n97 = invoke class="VI" method="FP.Close"(reference=w277, error in=w278) -> (error out=w279:errorcluster)  [unwired: 1 in, 2 out]
              }
            }
          }
          frame "Hidden", "Hide" {
            w280 = T1."Hidden" ("State")
            n98 = property class="VI"(reference=w286, error in=w285) -> (reference out=w283:refnum<vi>, error out=w284:errorcluster, "FP.State"=w282:T1)
            n99 = Not Equal?(x=w282, y=w280) -> (x != y?=w281:bool)
            n100 = case shown="True" w281 {
              tunnel: [w291 w292] -> w287
              tunnel: w284 -> [w290 w292]
              tunnel: w283 -> [w289 _]
              tunnel: w280 -> [w288 _]
              frame True {
                n101 = invoke class="VI" method="FP.Open"(reference=w289, error in=w290, "State"=w288) -> (error out=w291:errorcluster)  [unwired: 2 in, 4 out]
              }
              frame False {
              }
            }
          }
          frame "Minimize", "Minimized" {
            w293 = T1."Minimized" ("State")
            n102 = property class="VI"(reference=w299, error in=w298) -> (reference out=w296:refnum<vi>, error out=w297:errorcluster, "FP.State"=w295:T1)
            n103 = Not Equal?(x=w295, y=w293) -> (x != y?=w294:bool)
            n104 = case shown="True" w294 {
              tunnel: [w304 w305] -> w300
              tunnel: w297 -> [w303 w305]
              tunnel: w296 -> [w302 _]
              tunnel: w293 -> [w301 _]
              frame True {
                n105 = invoke class="VI" method="FP.Open"(reference=w302, error in=w303, "State"=w301) -> (error out=w304:errorcluster)  [unwired: 2 in, 4 out]
              }
              frame False {
              }
            }
          }
          frame "Maximize", "Maximized" {
            w306 = T1."Maximized" ("State")
            n106 = property class="VI"(reference=w312, error in=w311) -> (reference out=w309:refnum<vi>, error out=w310:errorcluster, "FP.State"=w308:T1)
            n107 = Not Equal?(x=w308, y=w306) -> (x != y?=w307:bool)
            n108 = case shown="True" w307 {
              tunnel: [w317 w318] -> w313
              tunnel: w310 -> [w316 w318]
              tunnel: w309 -> [w315 _]
              tunnel: w306 -> [w314 _]
              frame True {
                n109 = invoke class="VI" method="FP.Open"(reference=w315, error in=w316, "State"=w314) -> (error out=w317:errorcluster)  [unwired: 2 in, 4 out]
              }
              frame False {
              }
            }
          }
        }
      }
      frame "UI: Refresh Buttons" {
        # ":)"
        n110 = Unbundle By Name(w330) -> ("IsRunning?"=w320:bool)
        n111 = control-ref of="DAQ: Once"() -> (w329:refnum<vi>)
        n112 = control-ref of="Stop"() -> (w328:refnum<vi>)
        n113 = control-ref of="Start"() -> (w327:refnum<vi>)
        n114 = Not(x=w320) -> (.not. x?=w319:bool)
        n115 = Boolean To (0,1)(Boolean=w320) -> (0, 1=w326:i16)
        n116 = Boolean To (0,1)(Boolean=w319) -> (0, 1=w323:i16)
        n117 = Multiply(x=i16 2, y=w326) -> (x*y=w325:i16)
        n118 = Multiply(x=i16 2, y=w323) -> (x*y=w321:i16)
        n119 = property class="Bool"(reference=w329, "DisabledEnum"=w325) -> ()  [unwired: 1 in, 2 out]
        n120 = property class="Bool"(reference=w328, "DisabledEnum"=w321) -> ()  [unwired: 1 in, 2 out]
        n121 = property class="Bool"(reference=w327, "DisabledEnum"=w325) -> ()  [unwired: 1 in, 2 out]
      }
      frame "---------- Macro ----------" {
        # "#CSM \"Category Seperator\"\nDo not put any code in this frame."
        n122 = call <vilib>:"Add State(s) to Queue__JKI_lib_State_Machine.vi"("State(s) in (\"\")"=w336) -> ("States Out"=w335:string)  [unwired: 14 in]
      }
      frame "Macro: Initialize" {
        # "#CSM \"Macro: Initialize\"\nInitialization Macro (This is called once, when the VI starts)"
        n123 = call <vilib>:"Add State(s) to Queue__JKI_lib_State_Machine.vi"("State(s) in Front (\"\")"="Data: Initialize\nInitialize Core Data\nUI: Initialize\nData: Update Indicators", "State(s) in (\"\")"=w341) -> ("States Out"=w340:string)  [unwired: 13 in]
      }
      frame "Macro: DAQ Once" {
        n124 = call <vilib>:"Add State(s) to Queue__JKI_lib_State_Machine.vi"("State(s) in Front (\"\")"="DAQ: Initialize\nDAQ: Configure\nDAQ: Start\nData: Acquisite\nDAQ: Stop\nDAQ: Close\nUI: Refresh Buttons" ("State(s) in Front (\"\")"), "State(s) in (\"\")"=w343) -> ("States Out"=w344:string)  [unwired: 13 in]
      }
      frame "Macro: DAQ Continuous" {
        n125 = call "CSMLS - Define Loop State(s).vi"("States Out in"="DAQ: Initialize \nDAQ: Configure\nDAQ: Start\nUI: Refresh Buttons\nData: Acquisite\nDAQ: Continuous Check -><loop> \nDAQ: Stop\nDAQ: Close\nUI: Refresh Buttons -><end>" ("State(s) in Front (\"\")"), "Remaining States"=w348) -> ("States Out out"=w349:string)  [unwired: 13 in]
      }
      frame "Macro: Exit" {
        # "#CSM \"Macro: Exit\"\nExit Macro (This is called once, when the VI exits)"
        n126 = call <vilib>:"Add State(s) to Queue__JKI_lib_State_Machine.vi"("State(s) in (\"\")"="//Exit Sub-Modules ", "State(s) at Back (\"\")"="Data: Cleanup\nExit") -> ("States Out"=w355:string)  [unwired: 13 in]
        n127 = call "CSMLS - Add Exit State(s) with Loop Check.vi"("States Out in"=w355, "Remaining States"=w352) -> ("States Out out"=w358:string)  [unwired: 13 in]
      }
      frame "---------- API ----------" {
        # "#CSM \"Category Seperator\"\nDo not put any code in this frame."
      }
      frame "API: API1" {
        # "#CSM API Example\nCopy/Rename this case for your own API"
        # "#CSM Response\nConnect this to return the response of your API"
        # "#CSM >> Source CSM >>\nIf you need to tell who triggered this state , use this string. If it's this case itself, this string is \"\"."
        # "#CSM >> Arguments >>\nDeal with the parameter if any"
      }
      frame "API: API2" {
        # "#CSM API Example\nCopy/Rename this case for your own API"
        # "unpack Hex String  to Variant\nif complex parameter is needed."
        n128 = call "CSM - Convert HexStr to Data.vi"("HEX String"=w367) -> ()  [unwired: 7 in, 2 out]
        n129 = disable-structure shown="Disabled" {
          disable-tunnel: [w371 "API2 Response"] -> w366
          frame Disabled {
            # "pack variant to hexstr \nif complex response is needed."
            # "complex Response"
            n130 = call "CSM - Convert Data to HexStr.vi"() -> ("HEX String (0-9,A-F)"=w371:string)  [unwired: 9 in]
          }
          frame Enabled {
          }
        }
      }
      frame "---------- Internal ----------" {
        # "#CSM \"Category Seperator\"\nDo not put any code in this frame."
        n131 = call <vilib>:"Add State(s) to Queue__JKI_lib_State_Machine.vi"("State(s) in (\"\")"=w376) -> ("States Out"=w375:string)  [unwired: 14 in]
      }
      frame "Internal: button click" {
        # "#CSM \"Internal State\"\nThis category is used for holding internal states"
        n132 = call <vilib>:"Add State(s) to Queue__JKI_lib_State_Machine.vi"("State(s) in (\"\")"=w380) -> ("States Out"=w379:string)  [unwired: 14 in]
      }
      frame "Internal: pane resize" {
        # "#CSM \"Internal State\"\nThis category is used for holding internal states"
        n133 = call <vilib>:"Add State(s) to Queue__JKI_lib_State_Machine.vi"("State(s) in (\"\")"=w384) -> ("States Out"=w383:string)  [unwired: 14 in]
      }
      frame "Internal: Slide Change" {
        n134 = Bundle By Name(cluster=w387, "Center"="Center") -> (w386:T4)
      }
      frame "internal: generate low-priority error" {
      }
      frame "internal: generate high-priority error" {
      }
      frame "----------- daq ---------------" {
      }
      frame "DAQ: Initialize" {
      }
      frame "DAQ: Configure" {
      }
      frame "DAQ: Start" {
        n135 = Bundle By Name(cluster=w407, "IsRunning?"=TRUE) -> (w406:T4)
      }
      frame "Data: Acquisite" {
        n136 = Unbundle By Name(w411) -> ("Center"=w410:dbl)
        n137 = Random Number (0-1)() -> (number: 0 to 1=w413:dbl)
        n138 = Add(x=w413, y=w410) -> (x+y=→"Waveform Chart":dbl)
      }
      frame "DAQ: Continuous Check" {
        # "Loop timer"
        n139 = Wait (ms)(milliseconds to wait=u32 200) -> ()  [unwired: 1 out]
        n140 = call "CSMLS - Append Continuous State.vi"("Loop State(s) and Arguments"="Data: Acquisite", "Continous State"=w417, "Remaining States"=w419) -> ("States Out"=w420:string)  [unwired: 8 in]
        ">> Source CSM >>" <- w418
      }
      frame "DAQ: Break Continuous" {
        n141 = call "CSMLS - Remove Loop Tag to Break.vi"("Remaining States"=w425) -> ("States"=w424:string)  [unwired: 10 in]
      }
      frame "DAQ: Stop" {
        n142 = Bundle By Name(cluster=w430, "IsRunning?"=FALSE) -> (w429:T4)
      }
      frame "DAQ: Close" {
      }
    }
    "Remaining States" <- w72
  }
